vi "Find_time_to_half_max.vi"(2 "Slide":dbl(slide) scale=0.1..1.0, 9 "XY_pairs_in":cluster{"Array":dbl[], "Y":dbl[]}, 10 "Locations":dbl[](array[numeric]), 11 "Peaks_xy_in":cluster{"Array":dbl[], "Amplitudes":dbl[]}) -> (3 "points_to_half_max":dbl)   [LabVIEW 2015]
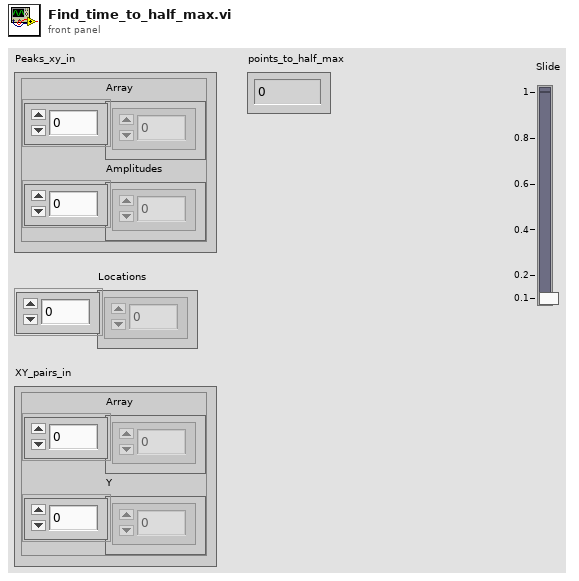
[diagram p1: front panel]
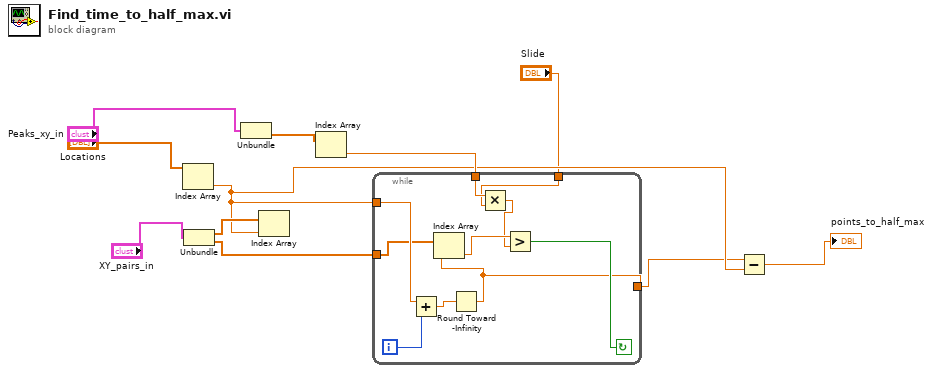
[diagram p0: block diagram]
diagram:
  n1 = Index Array(array="Locations") -> (element=w3:dbl)  [unwired: 1 in]
  n2 = Unbundle("XY_pairs_in") -> ("Array"=w11:dbl[], "Y"=w7:dbl[])
  n3 = Unbundle("Peaks_xy_in") -> ("Amplitudes"=w9:dbl[])  [unwired: 1 out]
  n4 = Index Array(array=w11, index=w3) -> ()  [unwired: 1 out]
  n5 = Index Array(array=w9) -> (element=w10:dbl)  [unwired: 1 in]
  n6 = while {
    tunnel: w7 -> [w19]
    tunnel: w3 -> [w21]
    tunnel: w10 -> [w14]
    tunnel: [w15] -> w2
    tunnel: "Slide" -> [w12]
    i -> [w20]
    stop <- w17 continue-if-true
    n7 = Add(x=w21, y=w20) -> (x+y=w16:dbl)
    n8 = Round Toward -Infinity(1:w16) -> (0:w15:dbl)
    n9 = Index Array(array=w19, index=w15) -> (element=w18:dbl)
    n10 = Multiply(x=w14, y=w12) -> (x*y=w13:dbl)
    n11 = Greater?(x=w18, y=w13) -> (0:w17:bool)
  }
  n12 = Subtract(x=w2, y=w3) -> (x-y=→"points_to_half_max":dbl)
